vi "optagefrekvenssignal0.2(SubVI).vi"() -> (1 "Max frequency":dbl, 2 "FFT power spectre":cluster{"f0":dbl, "df":dbl, "magnitude":dbl[]}(graph), 3 "Soundsignal":waveform(dbl)(graph))   [LabVIEW 2014]
uses:
  <vilib>/measure/maspectr.llb/FFT Power Spectrum and PSD for 1 Chan.vi
  <vilib>/measure/NI_MAPro.lvlib
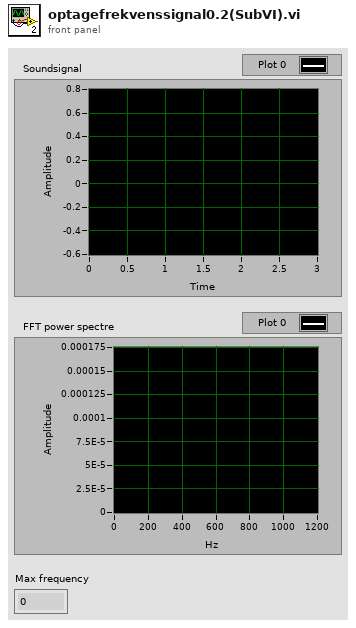
[diagram p1: front panel]
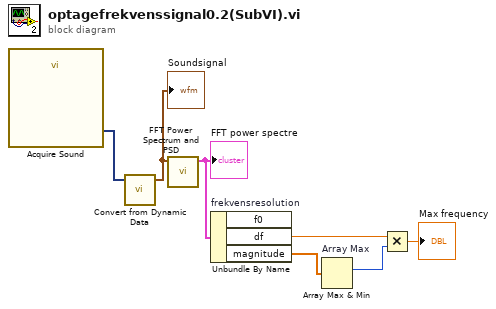
[diagram p0: block diagram]
diagram:
  n1 = call "Acquire Sound"() -> ("Data"=w5:dynamicdata)  [unwired: 18 in, 1 out]
  n2 = call "Convert from Dynamic Data"("Dynamic Data Type"=w5) -> ("Waveform"=w1:waveform(dbl))  [unwired: 3 in]
  "Soundsignal" <- w1
  n3 = call-poly <vilib>:"FFT Power Spectrum and PSD.vi"("time signal"=w1) -> ("Power Spectrum / PSD"=w2:cluster{"f0":dbl, "df":dbl, "magnitude":dbl[]})  [unwired: 7 in, 3 out]
  "FFT power spectre" <- w2
  n4 = Unbundle By Name "frekvensresolution"(w2) -> ("df"=w4:dbl, "magnitude"=w3:dbl[])  [unwired: 1 out]
  n5 = Array Max & Min "Array Max"(array=w3) -> (max index (indices)=w7:i32)  [unwired: 3 out]
  n6 = Multiply(x=w4, y=w7) -> (x*y=→"Max frequency":dbl)
